vi "Week5_Q3Real.vi"() -> ()   [LabVIEW 2021]
uses:
  <vilib>/LabVIEW Interface for Arduino/LabVIEW Interface for Arduino.lvlib
panel:
  in  "VISA resource":refnum<visa-resource-name>
  in  "Stop":bool
  in  "your answer":dbl
  in  "y":dbl
  in  "x":dbl
  in  "Select Operation":string(combo)
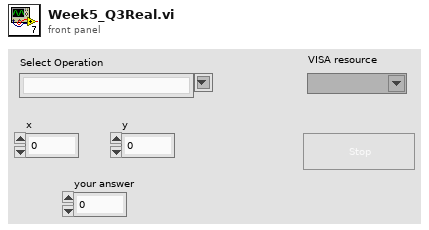
[diagram p1: front panel]
types:
  T1 = typedef "LabVIEW Interface for Arduino.lvlib/Arduino Resource.ctl" = cluster{"VISA resource":refnum<visa-resource-name>, "Board Type":T2, "Connection Type":enum8{"USB / Serial"}, "Bytes Per Packet (15)":u8}
  T2 = typedef "LabVIEW Interface for Arduino.lvlib/Board Type.ctl" = enum16{"Uno", "Dimuelanove w/Atmega 328", "Mega 2560"}
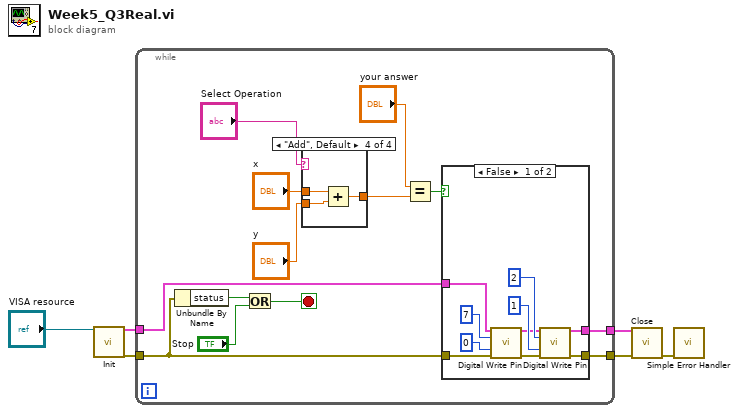
[diagram p0: block diagram]
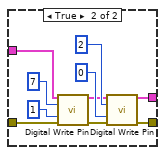
[diagram p2: hidden frame]
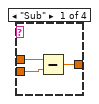
[diagram p3: hidden frame]
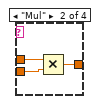
[diagram p4: hidden frame]
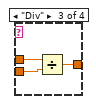
[diagram p5: hidden frame]
diagram:
  n1 = call <vilib>:"Init.vi"("VISA resource"="VISA resource") -> ("Arduino Resource"=w6:T1, "error out"=w4:errorcluster)  [unwired: 17 in]
  n2 = while {
    tunnel: w6 -> [w13]
    tunnel: [w12] -> w5
    tunnel: w4 -> [w7]
    tunnel: [w11] -> w3
    stop <- w8 stop-if-true
    n3 = Unbundle By Name(w7) -> ("status"=w10:bool)
    n4 = Or(x=w10, y="Stop") -> (x .or. y?=w8:bool)
    n5 = case shown="\"Add\", Default" "Select Operation" {
      tunnel: "x" -> [w42 w45 w48 w51]
      tunnel: "y" -> [w41 w44 w47 w50]
      tunnel: [w40 w43 w46 w49] -> w16
      frame "Sub" {
        n6 = Subtract(x=w42, y=w41) -> (x-y=w40:dbl)
      }
      frame "Mul" {
        n7 = Multiply(x=w45, y=w44) -> (x*y=w43:dbl)
      }
      frame "Div" {
        n8 = Divide(x=w48, y=w47) -> (x/y=w46:dbl)
      }
      frame "Add", Default {
        n9 = Add(x=w51, y=w50) -> (x+y=w49:dbl)
      }
    }
    n10 = Equal?(x="your answer", y=w16) -> (x = y?=w14:bool)
    n11 = case shown="False" w14 {
      tunnel: w13 -> [w25 w35]
      tunnel: [w23 w33] -> w12
      tunnel: w7 -> [w22 w32]
      tunnel: [w20 w30] -> w11
      frame False {
        n12 = call <vilib>:"Digital Write Pin.vi"("Arduino Resource"=w25, "Digital I/O Pin (0)"=u8 7, "Value (0)"=u8 0, "error in"=w22) -> ("Arduino Resource"=w24:T1, "error out"=w21:errorcluster)  [unwired: 10 in]
        n13 = call <vilib>:"Digital Write Pin.vi"("Arduino Resource"=w24, "Digital I/O Pin (0)"=u8 2, "Value (0)"=u8 1, "error in"=w21) -> ("Arduino Resource"=w23:T1, "error out"=w20:errorcluster)  [unwired: 10 in]
      }
      frame True {
        n14 = call <vilib>:"Digital Write Pin.vi"("Arduino Resource"=w35, "Digital I/O Pin (0)"=u8 7, "Value (0)"=u8 1, "error in"=w32) -> ("Arduino Resource"=w34:T1, "error out"=w31:errorcluster)  [unwired: 10 in]
        n15 = call <vilib>:"Digital Write Pin.vi"("Arduino Resource"=w34, "Digital I/O Pin (0)"=u8 2, "Value (0)"=u8 0, "error in"=w31) -> ("Arduino Resource"=w33:T1, "error out"=w30:errorcluster)  [unwired: 10 in]
      }
    }
  }
  n16 = call <vilib>:"Close.vi"("Arduino Resource"=w5, "error in"=w3) -> ("error out"=w2:errorcluster)  [unwired: 13 in]
  n17 = call <vilib>:"Simple Error Handler.vi"("error in (no error)"=w2) -> ()  [unwired: 4 in, 5 out]
